vi "CM_Packet_Encode_and_Decode_Test.vi"() -> ()   [LabVIEW 2017]
uses:
  Classes/ADCP.lvclass
panel:
  out "CM Packet output":T1
  in  "CM Packet input":T1
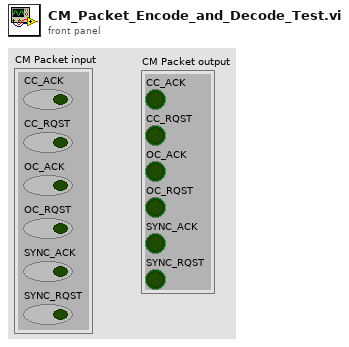
[diagram p1: front panel]
types:
  T1 = cluster{"CC_ACK":bool, "CC_RQST":bool, "OC_ACK":bool, "OC_RQST":bool, "SYNC_ACK":bool, "SYNC_RQST":bool}
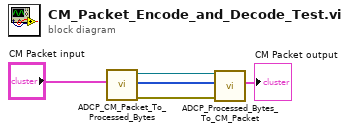
[diagram p0: block diagram]
diagram:
  n1 = call "ADCP_CM_Packet_To_Processed_Bytes.vi"("Connection Management"="CM Packet input") -> ("error out"=w4:errorcluster, "Processed Packet"=w3:u8[], "ADCP out"=w5:refnum<class "ADCP.lvclass">)  [unwired: 8 in]
  n2 = call "ADCP_Processed_Bytes_To_CM_Packet.vi"("error in (no error)"=w4, "Processed Packet Bytes"=w3, "ADCP In"=w5) -> ("CM Packet"=→"CM Packet output":T1)  [unwired: 6 in, 2 out]
